vi "STP Main.vi"(6 "Log Data?":bool, 8 "error in (no error)":errorcluster, 9 "CAN Init Data":T5={"XNET Interface"="CAN1", "Baud Rate"=500000, "CAN:Termination"=0, "Echo Transmit?"=FALSE, "scope (normal)"=0} {"scope (normal)" items=["Normal", "Session Only", "Interface Only", "Session Only Blocking"]; "CAN:Termination" items=["Off", "On"]; "Baud Rate" format="%.0p"}, 10 "CAN View Table":refnum<vi>, 11 "STP Input Data":T1={"TxID"=2042, "RxID"=2043, "CMD"=130, "RQ Data"=[], "+veResponseCode"=160, "ResponseTimeout (S)"=1.0} {"ResponseTimeout (S)" format="%#_13g"; "+veResponseCode" format="%x"; "CMD" items=["TSW_VERSION(130)"=130, "WAIT_EVENT(132)"=132, "SEQUENCER(133)"=133, "TSW_RESET(150)"=150, "CONFIG_ECU(151)"=151, "TEST_CORE (152)"=152, "TEST_WATCHDOG (153)"=153, "TEST_MONITORING (154)"=154, "READ_MEMORY (162)"=162, "WRITE_ERASE_MEMORY (164)"=164, "COMM_EXTERNAL (190)"=190, "COMM_INTERNAL (195)"=195, "GET_ANALOG_INPUT (210)"=210, "GET_DIGITAL_INPUT (211)"=211, "GET_FREQUENCY_INPUT (212)"=212, "TEST_INPUT_STRUCTURE (214)"=214, "GENERATE_OUTPUT_SIGNAL (220)"=220, "GENERATE_SYNCHRONIZED_OUTPUT_SIGNALS (221)"=221, "eDCU_Specific (250)"=250]; "RxID" format="%.0x"; "TxID" format="%.0x"}) -> (0 "error out":errorcluster, 2 "RequestTimeout?":bool, 3 "STP Output Data":T3)   [LabVIEW 2023, in "HardwareAbstractionLayer_LVOOP.lvlib" / "CAN Application Protocols Lib.lvlib" / "STP Protocol.lvclass"]
uses:
  STP Protocol.lvclass
  CAN Lib/CAN_class/Ctrls/CAN Init Ctrl.ctl
  <vilib>/xnet/xnet.llb/XNET Control Scope.ctl
  Ctrls/STP Output Data.ctl
  Ctrls/STP Error Cluster.ctl
  Ctrls/STP Input Data.ctl
  Ctrls/STP CMD.ctl
  CAN Lib/Control/CAN Table.ctl
  Ctrls/STP States.ctl
  CAN Lib/NI-XNET_class/NI-XNET.lvclass
  Ctrls/STP Loop Data.ctl
  STP Protocol.lvclass/STP Protocol.ctl
  <vilib>/xnet/xnet.llb/XNET Frame CAN.ctl
  <vilib>/xnet/xnet.llb/XNET Frame Type CAN.ctl
  Ctrls/TP Frame Type.ctl
  e618861d-f236-4a68-a3fc-cc1eaf20d10c.vi
  Teststand Steptypes/LTT_TeststandSteptypes.lvlib
  CAN Lib/CAN_class/CAN.lvclass
  CAN Lib/CAN HAL Lib.lvlib
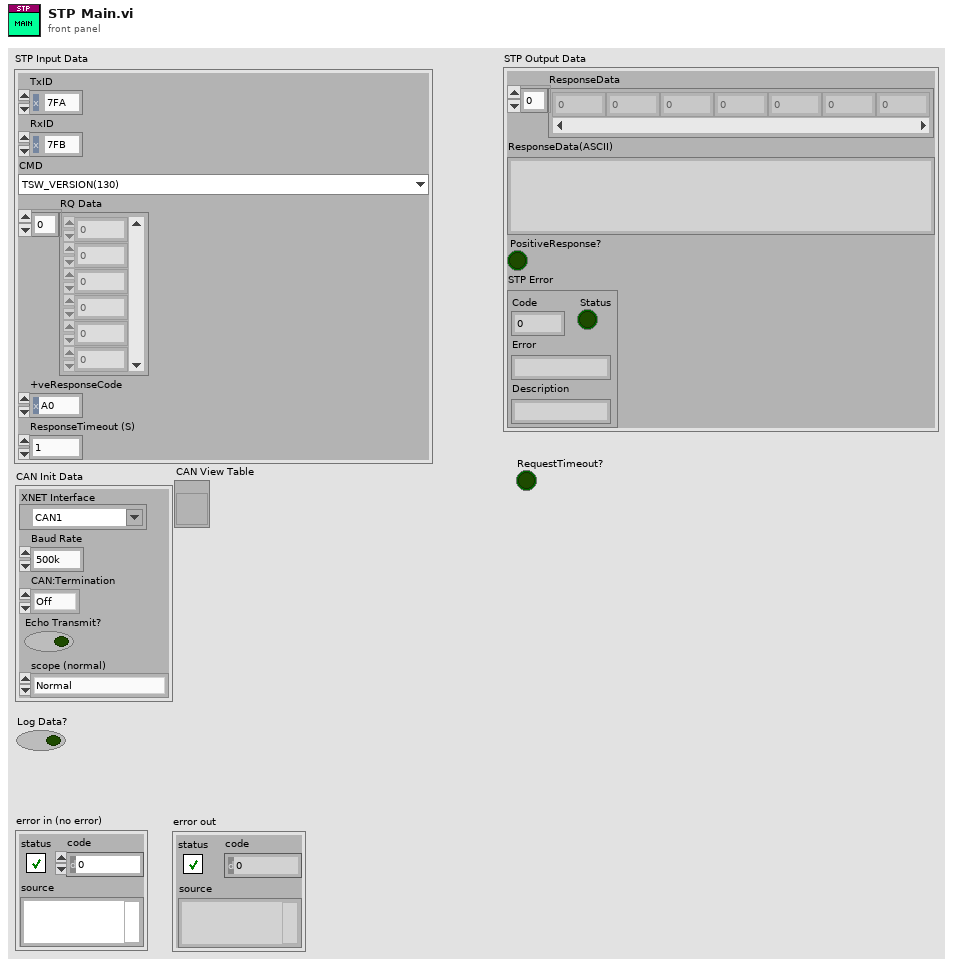
[diagram p1: front panel]
types:
  T1 = typedef "HardwareAbstractionLayer_LVOOP.lvlib/CAN Application Protocols Lib.lvlib/STP Protocol.lvclass/STP Input Data.ctl" = cluster{"TxID":u32, "RxID":u32, "CMD":T2, "RQ Data":u8[], "+veResponseCode":u8, "ResponseTimeout (S)":dbl}
  T2 = typedef "HardwareAbstractionLayer_LVOOP.lvlib/CAN Application Protocols Lib.lvlib/STP Protocol.lvclass/STP CMD.ctl" = u8
  T3 = typedef "HardwareAbstractionLayer_LVOOP.lvlib/CAN Application Protocols Lib.lvlib/STP Protocol.lvclass/STP Output Data.ctl" = cluster{"ResponseData":u8[], "ResponseData(ASCII)":string, "PositiveResponse?":bool, "STP Error":T4}
  T4 = typedef "HardwareAbstractionLayer_LVOOP.lvlib/CAN Application Protocols Lib.lvlib/STP Protocol.lvclass/STP Error Cluster.ctl" = cluster{"Status":bool, "Code":u8, "Error":string, "Description":string}
  T5 = typedef "HardwareAbstractionLayer_LVOOP.lvlib/CAN HAL Lib.lvlib/CAN.lvclass/CAN Init Ctrl.ctl" = cluster{"XNET Interface":refnum<k21>, "Baud Rate":u64, "CAN:Termination":u32, "Echo Transmit?":bool, "scope (normal)":T6}
  T6 = typedef "XNET Control Scope.ctl" = u32
  T7 = typedef "HardwareAbstractionLayer_LVOOP.lvlib/CAN Application Protocols Lib.lvlib/STP Protocol.lvclass/STP States.ctl" = enum16{"Init", "Send Request", "Check Ack", "Send TP Frames", "Send Flow Control Frame", "Check Response", "Read TP Data", "Return Data", "Return Positive Response", "Return Error Response", "Exit"}
  T8 = typedef "HardwareAbstractionLayer_LVOOP.lvlib/CAN Application Protocols Lib.lvlib/STP Protocol.lvclass/STP Loop Data.ctl" = cluster{"ResponseData":u8[], "DataSize(bytes)":u16, "ReceiveAllData?":bool, "PositiveResponse?":bool, "CosecutiveFrameID":fxp<+,4,4>, "#FrameToRead":i32}
  T9 = typedef "XNET Frame CAN.ctl" = cluster{"timestamp":timestamp, "payload":u8[], "identifier":u32, "type":T10, "extended?":bool, "echo?":bool}
  T10 = typedef "XNET Frame Type CAN.ctl" = u8
  T11 = typedef "HardwareAbstractionLayer_LVOOP.lvlib/CAN Application Protocols Lib.lvlib/STP Protocol.lvclass/TP Frame Type.ctl" = u8
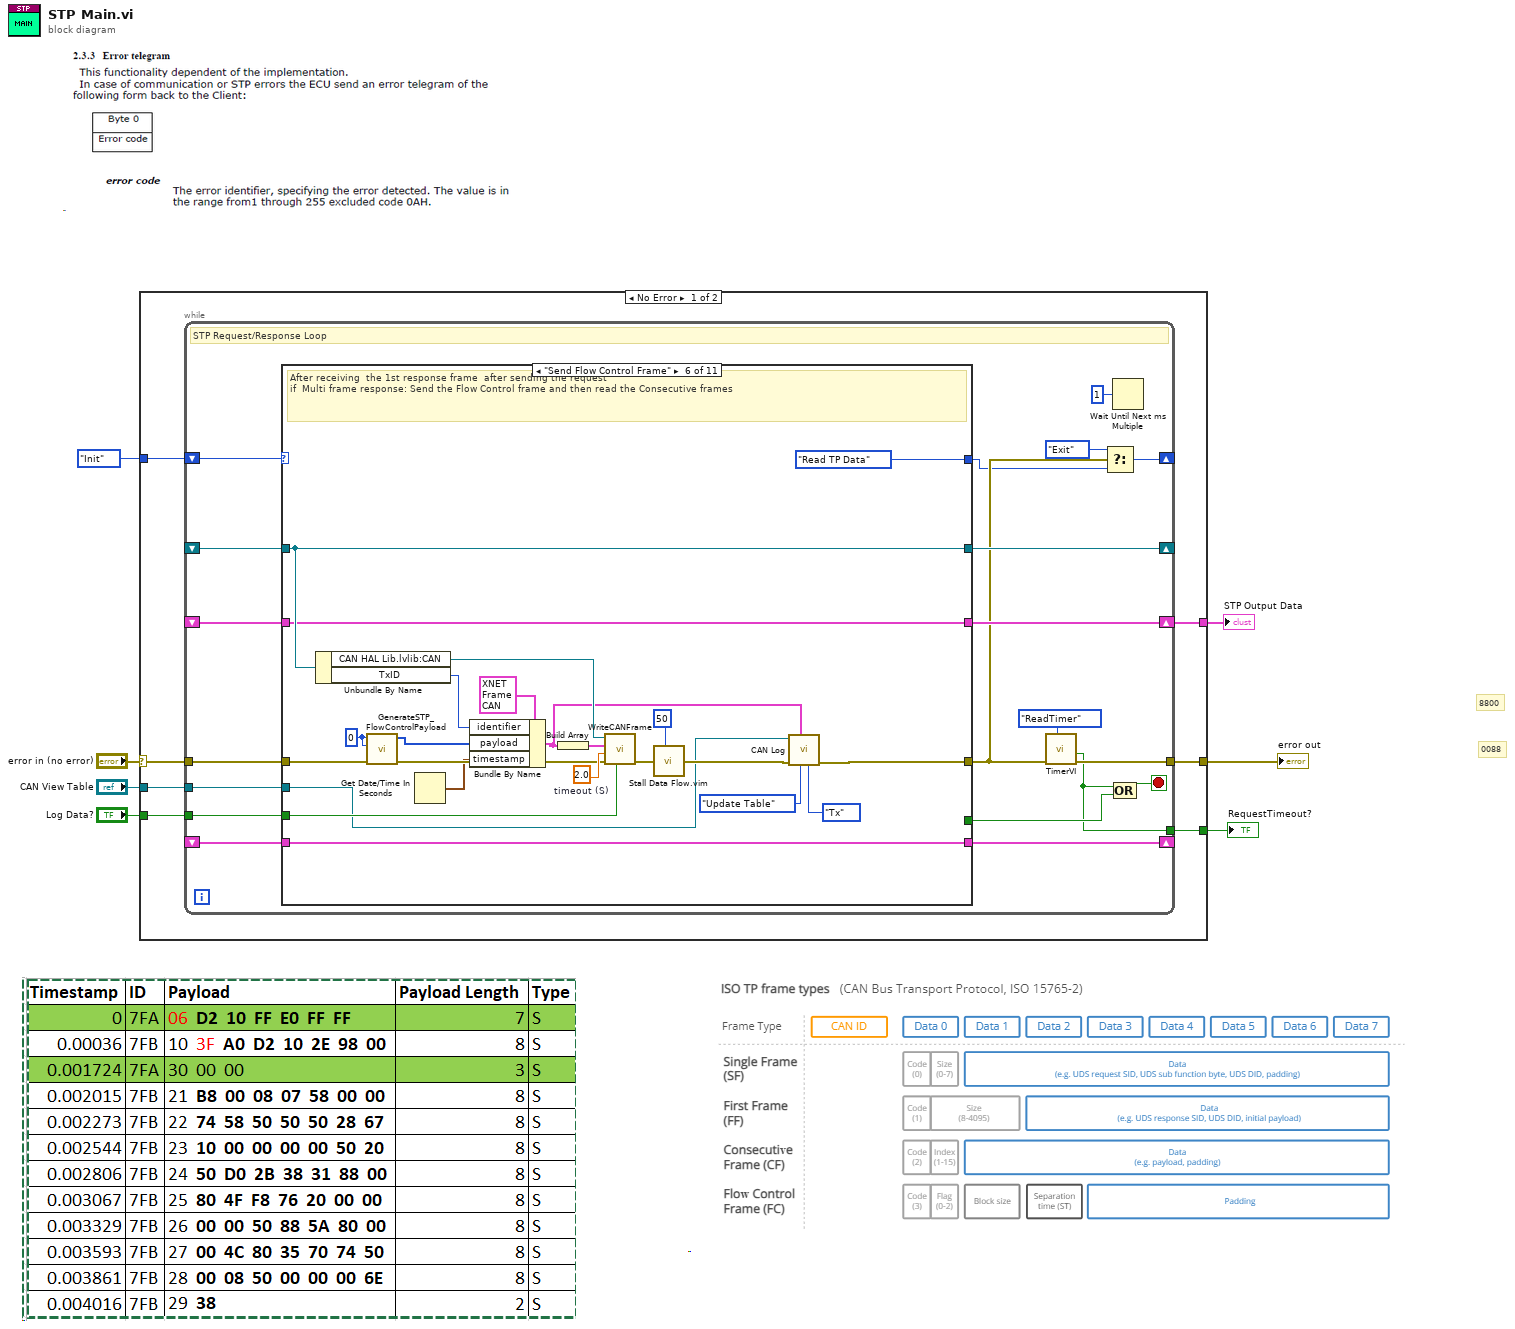
[diagram p0: block diagram]
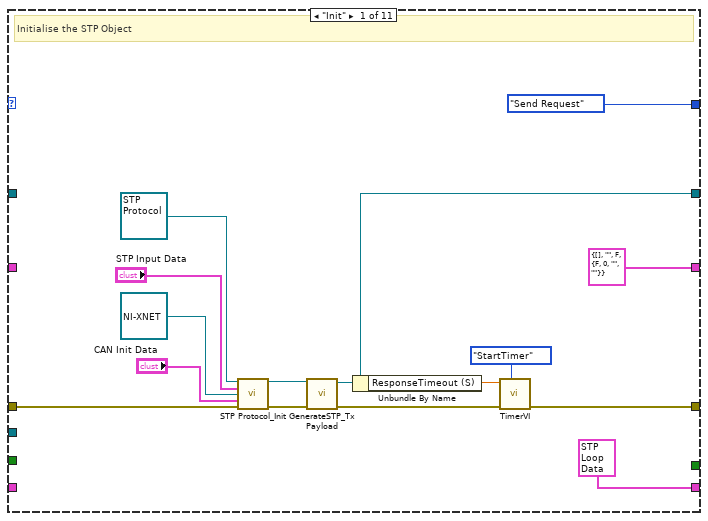
[diagram p2: hidden frame]
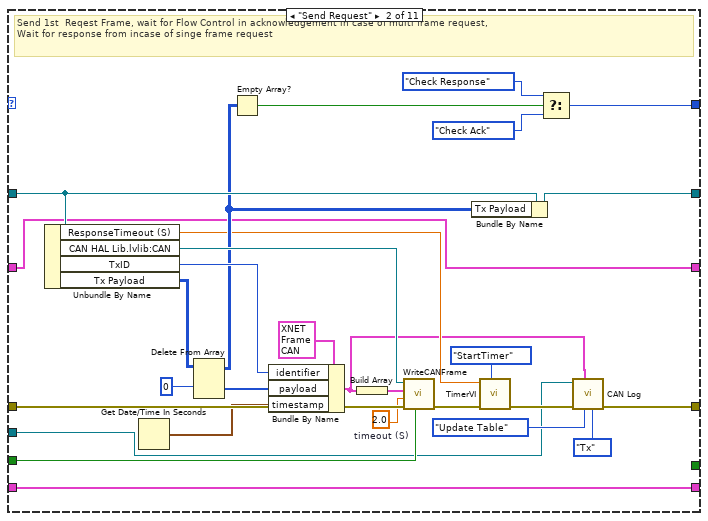
[diagram p3: hidden frame]
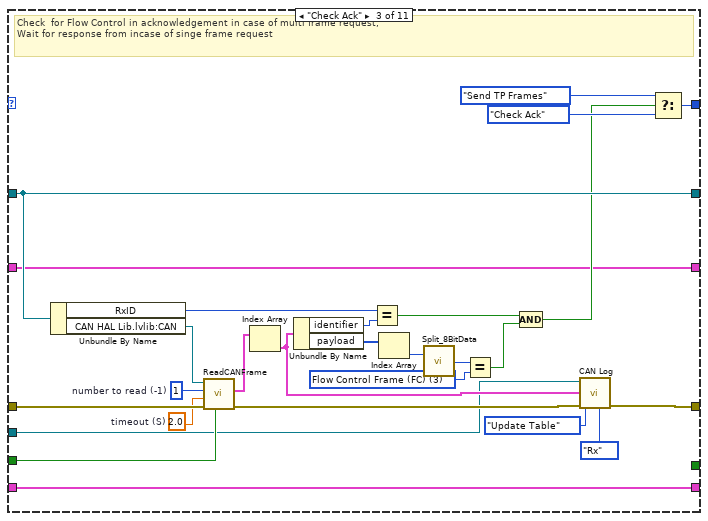
[diagram p4: hidden frame]
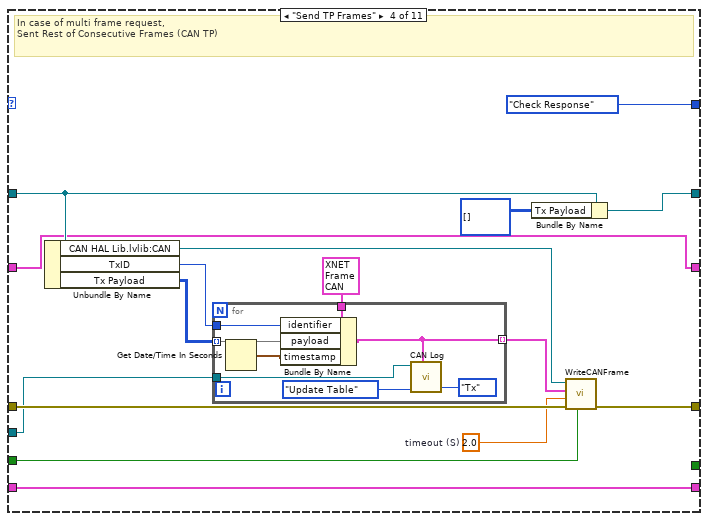
[diagram p5: hidden frame]
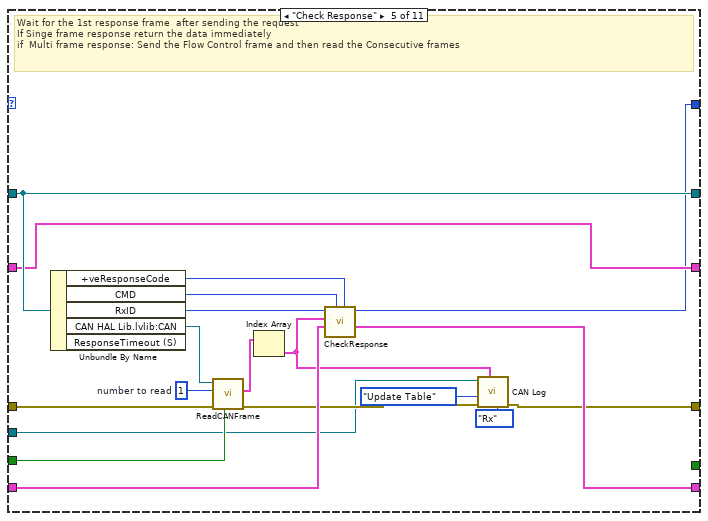
[diagram p6: hidden frame]
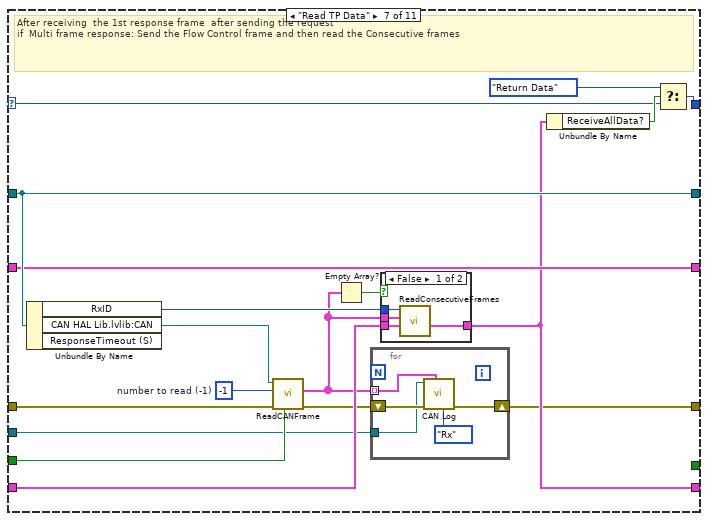
[diagram p7: hidden frame]
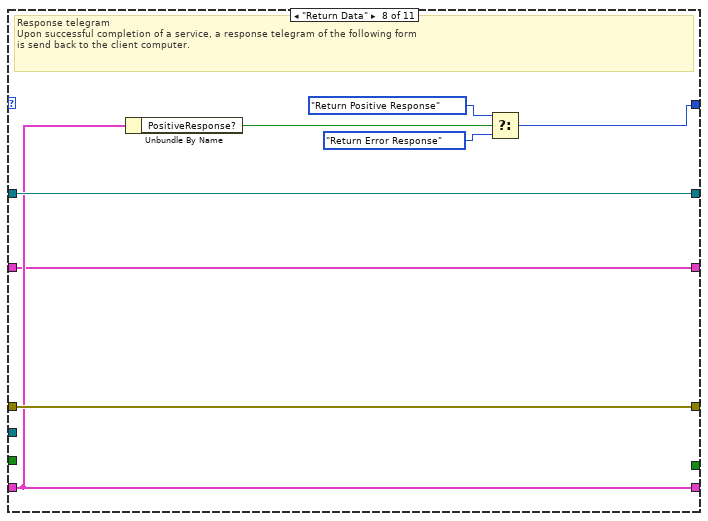
[diagram p9: hidden frame]
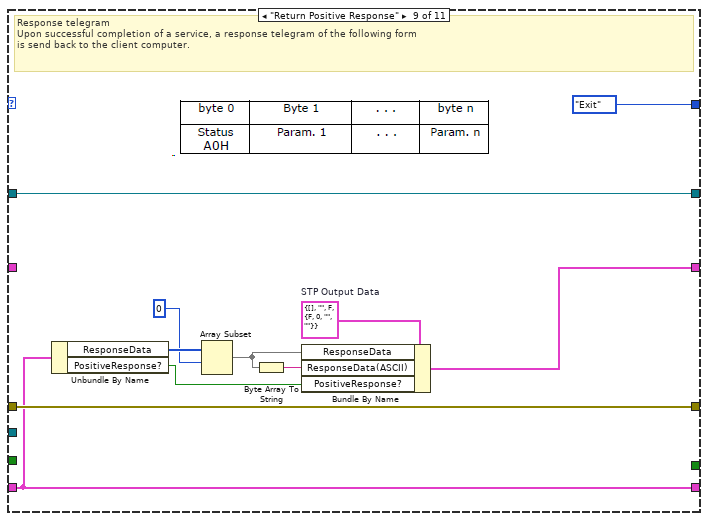
[diagram p10: hidden frame]
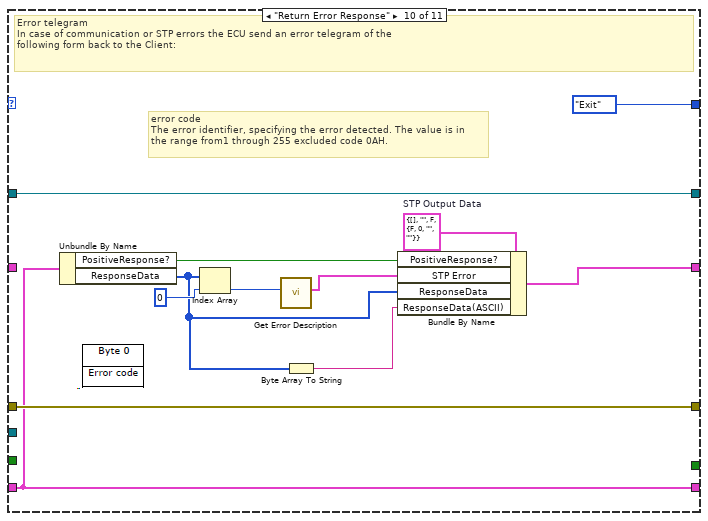
[diagram p11: hidden frame]
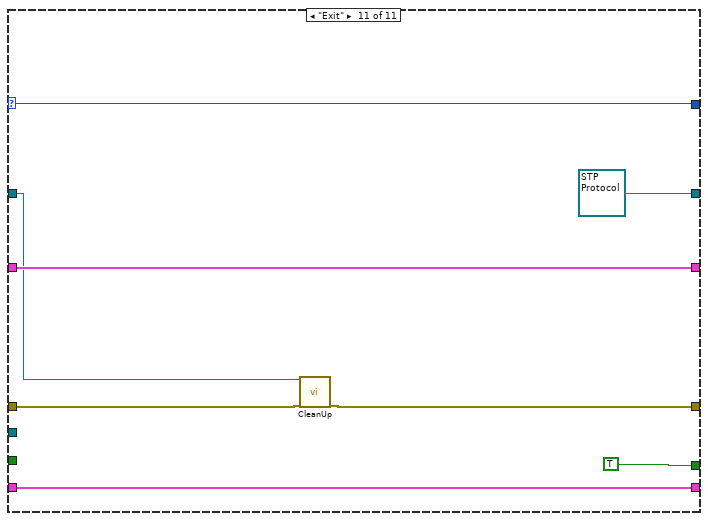
[diagram p12: hidden frame]
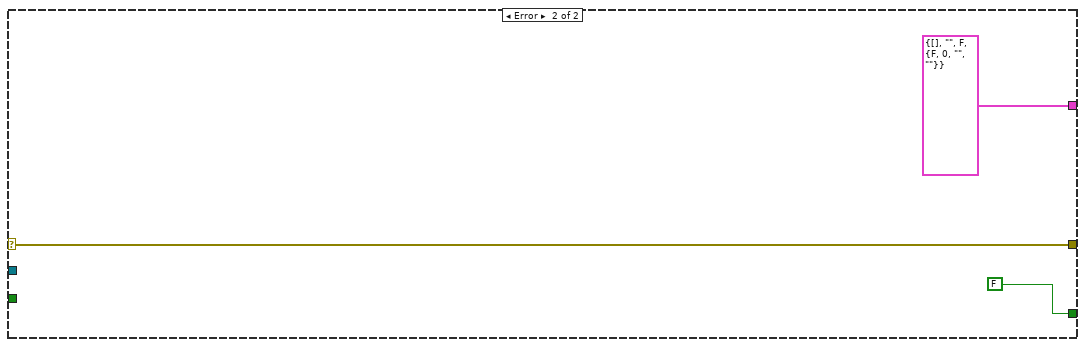
[diagram p13: hidden frame]
diagram:
  # "0088"
  # "8800"
  n1 = case shown="No Error" "error in (no error)" {
    selector: "error in (no error)" -> [w13 w241]
    tunnel: [w14 w241] -> w2
    tunnel: STP_States."Init" -> [w12 _]
    tunnel: [w11 T3 {"ResponseData"=[], "ResponseData(ASCII)"="", "PositiveResponse?"=FALSE, "STP Error"={"Status"=FALSE, "Code"=0, "Error"="", "Description"=""}} ("STP Output Data")] -> w5
    tunnel: [w10 FALSE ("TimeLapsed?")] -> w4
    tunnel: "Log Data?" -> [w9 _]
    tunnel: "CAN View Table" -> [w8 _]
    frame No Error {
      n2 = while {
        shift-right: [w34] -> _
        shift-left: _ -> [w33]
        shift-right: [w18] -> _
        shift-left: w12 -> [w32]
        tunnel: [w29] -> w14
        tunnel: w13 -> [w31]
        shift-right: [w27] -> _
        shift-left: _ -> [w26]
        tunnel: [w23] -> w10
        shift-right: [w24] -> w11
        shift-left: _ -> [w22]
        tunnel: w9 -> [w21]
        tunnel: w8 -> [w16]
        stop <- w30 stop-if-true
        # "STP Request/Response Loop"
        n3 = case shown="\"Send Flow Control Frame\"" w32 {
          selector: w32 -> [_ _ _ _ _ _ w184 _ _ _ w235]
          tunnel: [w37 w69 w105 w116 w148 w171 w189 w207 w218 w230 refnum<class "STP Protocol.lvclass"> refnum ("STP Protocol out")] -> w34
          tunnel: w33 -> [_ w78 w105 w121 w148 w171 w189 w207 w218 w230 w232]
          tunnel: [w38 w52 w80 w108 w137 w153 w176 w206 w217 w229 w231] -> w20
          tunnel: w31 -> [w44 w77 w104 w120 w147 w163 w188 w206 w217 w229 w233]
          tunnel: [STP_States."Send Request" w64 w100 STP_States."Check Response" w135 STP_States."Read TP Data" w182 w203 STP_States."Exit" STP_States."Exit" w235] -> w19
          tunnel: [T8 {"ResponseData"=[], "DataSize(bytes)"=0, "ReceiveAllData?"=FALSE, "PositiveResponse?"=FALSE, "CosecutiveFrameID"=1.0, "#FrameToRead"=0} ("STP Loop Data Out") w60 w87 w111 w145 w164 w179 w201 w215 w227 w238] -> w27
          tunnel: w26 -> [_ w60 w87 w111 w144 w164 w178 w201 w215 w227 w238]
          tunnel: [_ _ _ _ _ _ _ _ _ _ TRUE] -> w25
          tunnel: [T3 {"ResponseData"=[], "ResponseData(ASCII)"="", "PositiveResponse?"=FALSE, "STP Error"={"Status"=FALSE, "Code"=0, "Error"="", "Description"=""}} ("STP Output Data") w56 w85 w109 w139 w155 w180 w200 w212 w225 w234] -> w24
          tunnel: w22 -> [_ w56 w85 w109 w139 w155 w180 w200 _ _ w234]
          tunnel: w21 -> [_ w58 w86 w110 w140 w157 w181 _ _ _ _]
          tunnel: w16 -> [_ w50 w79 w106 w136 w150 w175 _ _ _ _]
          frame "Init" {
            # "Initialise the STP Object"
            n4 = call "STP Protocol_Init.vi"("object in"=refnum<class "STP Protocol.lvclass"> refnum ("STP Protocol in"), "Init Data"="STP Input Data", "CAN HAL Lib.lvlib:NI-XNET"=refnum<class "NI-XNET.lvclass"> refnum, "CAN Init Data"="CAN Init Data", "error in (no error)"=w44) -> ("object out"=w49:refnum<class "STP Protocol.lvclass">, "error out"=w48:errorcluster)  [unwired: 9 in]
            n5 = call "GenerateSTP_Tx Payload.vi"("error in (no error)"=w48, "STP Protocol in"=w49) -> ("error out"=w39:errorcluster, "STP Protocol out"=w37:refnum<class "STP Protocol.lvclass">)  [unwired: 8 in]
            n6 = Unbundle By Name(w37) -> ("ResponseTimeout (S)"=w36:dbl)
            n7 = call "TimerVI.vi"("TimerAction(Read)"=enum16{"StartTimer", "ReadTimer"}."StartTimer", "error in (no error)"=w39, "TargetTime(mS)"=w36) -> ("error out"=w38:errorcluster)  [unwired: 6 in, 2 out]
          }
          frame "Send Request" {
            w61 = 2.0  # timeout (S)
            # "Send 1st  Reqest Frame, wait for Flow Control in acknowledgement in case of multi frame request,\nWait for response from incase of singe frame request"
            n8 = Unbundle By Name(w78) -> ("ResponseTimeout (S)"=w59:dbl, "CAN HAL Lib.lvlib:CAN"=w76:refnum<class "NI-XNET.lvclass">, "TxID"=w74:u32, "Tx Payload"=w73:u8[][])
            n9 = Get Date/Time In Seconds() -> (seconds since 1Jan1904=w57:timestamp)
            n10 = Delete From Array(array=w73, index (row)=0) -> (deleted portion=w71:u8[], array with subset deleted=w68:u8[][])  [unwired: 2 in]
            n11 = Empty Array?(array=w68) -> (empty?=w67:bool)
            n12 = Bundle By Name(cluster=T9 {"timestamp"=timestamp(0 s since 1904-01-01), "payload"=[], "identifier"=0, "type"=0, "extended?"=FALSE, "echo?"=FALSE} ("CAN frame"), "identifier"=w74, "payload"=w71, "timestamp"=w57) -> (w51:T9)
            n13 = Build Array(w51) -> (w70:T9[])
            n14 = call-dynamic "WriteCANFrame.vi"("Log Data?"=w58, "error in (no error)"=w77, "timeout (10)"=w61, "data"=w70, "NI-XNET in"=w76) -> ("error out"=w63:errorcluster)  [unwired: 5 in, 1 out]
            n15 = Bundle By Name(cluster=w78, "Tx Payload"=w68) -> (w69:refnum<class "STP Protocol.lvclass">)
            n16 = call "TimerVI.vi"("TimerAction(Read)"=enum16{"StartTimer", "ReadTimer"}."StartTimer", "error in (no error)"=w63, "TargetTime(mS)"=w59) -> ("error out"=w53:errorcluster)  [unwired: 6 in, 2 out]
            n17 = Select(t=STP_States."Check Response", s=w67, f=STP_States."Check Ack") -> (s? t:f=w64:T7)
            n18 = call "CAN Log.vi"("TX/RX?"=enum16{"Tx", "Rx"}."Tx", "Action"=enum16{"Update Table", "Clear Table"}."Update Table", "CAN frame"=w51, "error in (no error)"=w53, "CAN View Table"=w50) -> ("error out"=w52:errorcluster)  [unwired: 6 in]
          }
          frame "Check Ack" {
            w88 = 1  # number to read (-1)
            w89 = 2.0  # timeout (S)
            w94 = T11 3 items=["Single Frame (SF)", "First Frame (SF)", "Consecutive Frame (CF)", "Flow Control Frame (FC)"] ("Ring")
            # "Check  for Flow Control in acknowledgement in case of multi frame request,\nWait for response from incase of singe frame request"
            n19 = Unbundle By Name(w105) -> ("RxID"=w97:u32, "CAN HAL Lib.lvlib:CAN"=w103:refnum<class "NI-XNET.lvclass">)
            n20 = call-dynamic "ReadCANFrame.vi"("Log Data?"=w86, "error in (no error)"=w104, "timeout (0)"=w89, "number to read (-1)"=w88, "NI-XNET in"=w103) -> ("error out"=w81:errorcluster, "data"=w99:T9[])  [unwired: 4 in, 1 out]
            n21 = Index Array(array=w99) -> (element=w82:T9)  [unwired: 1 in]
            n22 = Unbundle By Name(w82) -> ("identifier"=w98:u32, "payload"=w96:u8[])
            n23 = Equal?(x=w97, y=w98) -> (x = y?=w92:bool)
            n24 = Index Array(array=w96) -> (element=w95:u8)  [unwired: 1 in]
            n25 = call "Split_8BitData.vi"("x"=w95) -> ("lo(x)"=w93:u8)  [unwired: 17 in, 1 out]
            n26 = Equal?(x=w93, y=w94) -> (x = y?=w91:bool)
            n27 = Compound Arithmetic op=AND(w92, w91) -> (w90:bool)
            n28 = call "CAN Log.vi"("TX/RX?"=enum16{"Tx", "Rx"}."Rx", "Action"=enum16{"Update Table", "Clear Table"}."Update Table", "CAN frame"=w82, "error in (no error)"=w81, "CAN View Table"=w79) -> ("error out"=w80:errorcluster)  [unwired: 6 in]
            n29 = Select(t=STP_States."Send TP Frames", s=w90, f=STP_States."Check Ack") -> (s? t:f=w100:T7)
          }
          frame "Send TP Frames" {
            w115 = 2.0  # timeout (S)
            # "In case of multi frame request,\nSent Rest of Consecutive Frames (CAN TP)"
            n30 = Unbundle By Name(w121) -> ("CAN HAL Lib.lvlib:CAN"=w119:refnum<class "NI-XNET.lvclass">, "TxID"=w117:u32, "Tx Payload"=w112:u8[][])
            n31 = for {
              tunnel: T9 {"timestamp"=timestamp(0 s since 1904-01-01), "payload"=[], "identifier"=0, "type"=0, "extended?"=FALSE, "echo?"=FALSE} ("CAN frame") -> [w129]
              tunnel: w117 -> [w128]
              tunnel: w112 -> [w127] mode=indexing
              tunnel: [w124] -> w107 mode=indexing
              tunnel: w106 -> [w125]
              n32 = Get Date/Time In Seconds() -> (seconds since 1Jan1904=w126:timestamp)
              n33 = Bundle By Name(cluster=w129, "identifier"=w128, "payload"=w127, "timestamp"=w126) -> (w124:T9)
              n34 = call "CAN Log.vi"("TX/RX?"=enum16{"Tx", "Rx"}."Tx", "Action"=enum16{"Update Table", "Clear Table"}."Update Table", "CAN frame"=w124, "CAN View Table"=w125) -> ()  [unwired: 7 in, 1 out]
            }
            n35 = Bundle By Name(cluster=w121, "Tx Payload"=u8[][] []) -> (w116:refnum<class "STP Protocol.lvclass">)
            n36 = call-dynamic "WriteCANFrame.vi"("Log Data?"=w110, "error in (no error)"=w120, "timeout (10)"=w115, "data"=w107, "NI-XNET in"=w119) -> ("error out"=w108:errorcluster)  [unwired: 5 in, 1 out]
          }
          frame "Check Response" {
            w130 = 1  # number to read
            # "Wait for the 1st response frame  after sending the request\nIf Singe frame response return the data immediately\nif  Multi frame response: Send the Flow Control frame and then read the Consecutive frames"
            n37 = Unbundle By Name(w148) -> ("+veResponseCode"=w141:u8, "CMD"=w142:T2, "RxID"=w143:u32, "CAN HAL Lib.lvlib:CAN"=w146:refnum<class "NI-XNET.lvclass">)  [unwired: 1 out]
            n38 = call-dynamic "ReadCANFrame.vi"("Log Data?"=w140, "error in (no error)"=w147, "number to read (-1)"=w130, "NI-XNET in"=w146) -> ("error out"=w138:errorcluster, "data"=w132:T9[])  [unwired: 5 in, 1 out]
            n39 = Index Array(array=w132) -> (element=w131:T9)  [unwired: 1 in]
            n40 = call "CheckResponse.vi"("+veResponseCode"=w141, "STP CMD"=w142, "STP Loop Data In"=w144, "Rx CAN frame"=w131, "RxID"=w143) -> ("STP Loop Data Out"=w145:T8, "STP_NextState"=w135:T7)  [unwired: 4 in, 1 out]
            n41 = call "CAN Log.vi"("TX/RX?"=enum16{"Tx", "Rx"}."Rx", "Action"=enum16{"Update Table", "Clear Table"}."Update Table", "CAN frame"=w131, "error in (no error)"=w138, "CAN View Table"=w136) -> ("error out"=w137:errorcluster)  [unwired: 6 in]
          }
          frame "Send Flow Control Frame" {
            w161 = u8 0 ("BlockSize(BS)")
            w165 = 2.0  # timeout (S)
            # "After receiving  the 1st response frame  after sending the request\nif  Multi frame response: Send the Flow Control frame and then read the Consecutive frames"
            n42 = Unbundle By Name(w171) -> ("CAN HAL Lib.lvlib:CAN"=w159:refnum<class "NI-XNET.lvclass">, "TxID"=w169:u32)
            n43 = call "GenerateSTP_FlowControlPayload.vi"("error in (no error)"=w163, "SeperationTime(ST)"=w161, "BlockSize(BS)"=w161) -> ("error out"=w162:errorcluster, "Flow Control Payload"=w160:u8[])  [unwired: 7 in]
            n44 = Get Date/Time In Seconds() -> (seconds since 1Jan1904=w156:timestamp)
            n45 = Bundle By Name(cluster=T9 {"timestamp"=timestamp(0 s since 1904-01-01), "payload"=[], "identifier"=0, "type"=0, "extended?"=FALSE, "echo?"=FALSE} ("CAN frame"), "identifier"=w169, "payload"=w160, "timestamp"=w156) -> (w149:T9)
            n46 = Build Array(w149) -> (w168:T9[])
            n47 = call-dynamic "WriteCANFrame.vi"("Log Data?"=w157, "error in (no error)"=w162, "timeout (10)"=w165, "data"=w168, "NI-XNET in"=w159) -> ("error out"=w166:errorcluster)  [unwired: 5 in, 1 out]
            n48 = call "Stall Data Flow.vim"("value in"=w166, "milliseconds to wait"=u32 50) -> ("value out"=w154:errorcluster)  [unwired: 1 out]
            n49 = call "CAN Log.vi"("TX/RX?"=enum16{"Tx", "Rx"}."Tx", "Action"=enum16{"Update Table", "Clear Table"}."Update Table", "CAN frame"=w149, "error in (no error)"=w154, "CAN View Table"=w150) -> ("error out"=w153:errorcluster)  [unwired: 6 in]
          }
          frame "Read TP Data" {
            w174 = -1  # number to read (-1)
            # "After receiving  the 1st response frame  after sending the request\nif  Multi frame response: Send the Flow Control frame and then read the Consecutive frames"
            n50 = Unbundle By Name(w189) -> ("RxID"=w186:u32, "CAN HAL Lib.lvlib:CAN"=w187:refnum<class "NI-XNET.lvclass">)  [unwired: 1 out]
            n51 = call-dynamic "ReadCANFrame.vi"("Log Data?"=w181, "error in (no error)"=w188, "number to read (-1)"=w174, "NI-XNET in"=w187) -> ("error out"=w177:errorcluster, "data"=w172:T9[])  [unwired: 5 in, 1 out]
            n52 = Empty Array?(array=w172) -> (empty?=w173:bool)
            n53 = for {
              tunnel: w175 -> [w197]
              shift-right: [w198] -> w176
              shift-left: w177 -> [w199]
              tunnel: w172 -> [w195] mode=indexing
              n54 = call "CAN Log.vi"("TX/RX?"=enum16{"Tx", "Rx"}."Rx", "CAN frame"=w195, "error in (no error)"=w199, "CAN View Table"=w197) -> ("error out"=w198:errorcluster)  [unwired: 7 in]
            }
            n55 = case shown="False" w173 {
              tunnel: w186 -> [w193 _]
              tunnel: [w192 w194] -> w179
              tunnel: w178 -> [w191 w194]
              tunnel: w172 -> [w190 _]
              frame False {
                n56 = call "ReadConsecutiveFrames.vi"("STP Loop Data In"=w191, "CAN Data"=w190, "RxID"=w193) -> ("STP Loop Data Out"=w192:T8)  [unwired: 8 in]
              }
              frame True {
              }
            }
            n57 = Unbundle By Name(w179) -> ("ReceiveAllData?"=w185:bool)
            n58 = Select(t=STP_States."Return Data", s=w185, f=w184) -> (s? t:f=w182:T7)
          }
          frame "Return Data" {
            # "Response telegram\nUpon successful completion of a service, a response telegram of the following form\nis send back to the client computer."
            n59 = Unbundle By Name(w201) -> ("PositiveResponse?"=w205:bool)
            n60 = Select(t=STP_States."Return Positive Response", s=w205, f=STP_States."Return Error Response") -> (s? t:f=w203:T7)
          }
          frame "Return Positive Response" {
            w213 = T3 {"ResponseData"=[], "ResponseData(ASCII)"="", "PositiveResponse?"=FALSE, "STP Error"={"Status"=FALSE, "Code"=0, "Error"="", "Description"=""}}  # STP Output Data
            # "Response telegram\nUpon successful completion of a service, a response telegram of the following form\nis send back to the client computer."
            n61 = Unbundle By Name(w215) -> ("ResponseData"=w211:u8[], "PositiveResponse?"=w214:bool)
            n62 = Array Subset(array=w211, index=0) -> (w208:u8[])  [unwired: 1 in]
            n63 = Byte Array To String(unsigned byte array=w208) -> (string=w209:string)
            n64 = Bundle By Name(cluster=w213, "ResponseData"=w208, "ResponseData(ASCII)"=w209, "PositiveResponse?"=w214) -> (w212:T3)
          }
          frame "Return Error Response" {
            w226 = T3 {"ResponseData"=[], "ResponseData(ASCII)"="", "PositiveResponse?"=FALSE, "STP Error"={"Status"=FALSE, "Code"=0, "Error"="", "Description"=""}}  # STP Output Data
            # "error code\nThe error identifier, specifying the error detected. The value is in\nthe range from1 through 255 excluded code 0AH."
            # "Error telegram\nIn case of communication or STP errors the ECU send an error telegram of the\nfollowing form back to the Client:"
            n65 = Unbundle By Name(w227) -> ("PositiveResponse?"=w224:bool, "ResponseData"=w220:u8[])
            n66 = Index Array(array=w220, index=0) -> (element=w222:u8)
            n67 = call "Get Error Description.vi"("Code"=w222) -> ("STP Error"=w221:T4)  [unwired: 10 in]
            n68 = Byte Array To String(unsigned byte array=w220) -> (string=w219:string)
            n69 = Bundle By Name(cluster=w226, "PositiveResponse?"=w224, "STP Error"=w221, "ResponseData"=w220, "ResponseData(ASCII)"=w219) -> (w225:T3)
          }
          frame "Exit" {
            n70 = call-dynamic "CleanUp.vi"("object in"=w232, "error in (no error)"=w233) -> ("error out"=w231:errorcluster)  [unwired: 16 in, 1 out]
          }
        }
        n71 = call "TimerVI.vi"("TimerAction(Read)"=enum16{"StartTimer", "ReadTimer"}."ReadTimer", "error in (no error)"=w20) -> ("error out"=w29:errorcluster, "TimeLapsed?"=w23:bool)  [unwired: 7 in, 1 out]
        n72 = Select(t=STP_States."Exit", s=w20, f=w19) -> (s? t:f=w18:T7)
        n73 = Wait Until Next ms Multiple(millisecond multiple=u32 1) -> ()  [unwired: 1 out]
        n74 = Compound Arithmetic op=OR(w23, w25) -> (w30:bool)
      }
    }
    frame Error {
    }
  }
  "error out" <- w2
  "STP Output Data" <- w5
  "RequestTimeout?" <- w4
